vi "Copy InstrumentStudio Plug-In Main VI.vi"(0 "configuration":T1, 5 "Plugin Library Path":path, 11 "error in":errorcluster) -> (4 "IS Plugin Main VI Path":path, 15 "error out":errorcluster)   [LabVIEW 2021, in "InstrumentStudio Plug-In Editor.lvlib"]
uses:
  InstrumentStudio Plug-In Editor.lvlib
  controls/Data Holder.ctl
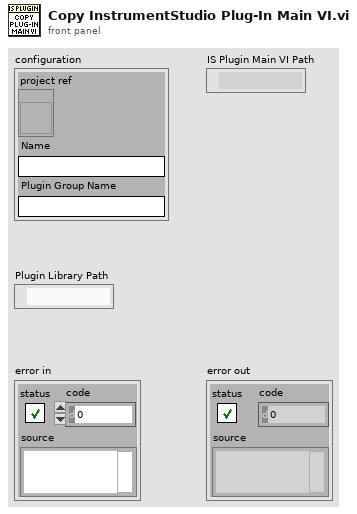
[diagram p1: front panel]
types:
  T1 = typedef "InstrumentStudio Plug-In Editor.lvlib/Data Holder.ctl" = cluster{"project ref":refnum<vi>, "Name":string, "Plugin Group Name":string}
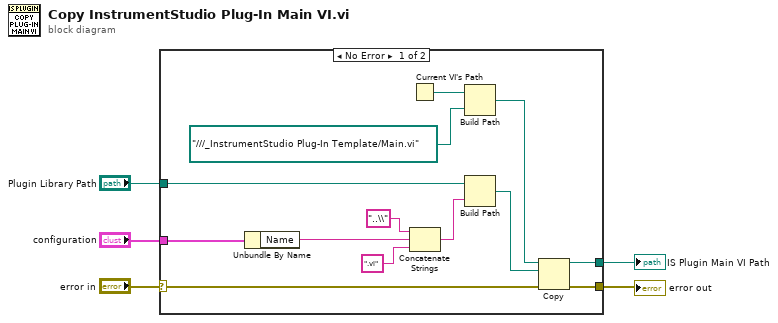
[diagram p0: block diagram]
diagram:
  n1 = case shown="No Error" "error in" {
    selector: "error in" -> [w18 w19]
    tunnel: [w15 w19] -> w5
    tunnel: "Plugin Library Path" -> [w16 _]
    tunnel: "configuration" -> [w6 _]
    tunnel: [w7 _] -> w1
    frame No Error {
      n2 = Unbundle By Name(w6) -> ("Name"=w13:string)
      n3 = Current VI's Path() -> (path=w10:path)
      n4 = Concatenate Strings("..\\" ("string"), w13, ".vi" ("string")) -> (w9:string)
      n5 = Build Path(base path=w10, name or relative path=path "../../../_InstrumentStudio Plug-In Template/Main.vi") -> (appended path=w14:path)
      n6 = Build Path(base path=w16, name or relative path=w9) -> (appended path=w17:path)
      n7 = Copy(8:w18, 10:w17, 11:w14) -> (0:w15:errorcluster, 3:w7:path)  [unwired: 2 in, 1 out]
    }
    frame Error {
    }
  }
  "error out" <- w5
  "IS Plugin Main VI Path" <- w1
